vi "_LC Send Command.vi"(4 "VialNumber":i16=1, 5 "SparkParameters":T1={"PlatePosition"=1, "SampleColumn"=97, "TrayType"=3}, 6 "RackType":i32(ring) items=["RackSVial"=0, "RackLVial"=1, "RackSPeltier"=2, "RackLPeltier"=3, "RackSingleMTP"=4, "RackDualMTP"=5, "RackLL"=6, "Rack2"=17, "Rack1"=18, "Rack3"=19, "Rack4"=20, "Rack5"=21, "Rack6"=22, "Rack7"=23, "Rack12"=33, "Rack11"=34, "Rack13"=35, "Rack14"=36, "Rack15"=37, "Rack16"=38, "Rack17"=39, "Rack_2010A_15Standard"=49, "Rack_2010A_1Standard"=50, "Rack_2010A_4Standard"=51, "Rack_2010A_MTP96Standard"=52, "Rack_2010A_MTP384Standard"=53, "Rack_2010A_DW96Standard"=54, "Rack_2010A_DW384Standard"=55, "Rack_2010A_15Cooled"=65, "Rack_2010A_1Cooled"=66, "Rack_2010A_4Cooled"=67, "Rack_2010A_MTP96Cooled"=68, "Rack_2010A_MTP384Cooled"=69, "Rack_2010A_DW96Cooled"=70, "Rack_2010A_DW384Cooled"=71, "Rack_20A_RACKCHANGER"=72, "Rack12A"=80, "Rack14A"=81, "Rack8"=82, "Rack9"=83, "Rack10"=84, "Rack14DDW"=85, "Rack5U"=86, "Rack4U"=87, "ControlRack"=119, "RackNone"=136, "RackUnknown"=153], 7 "InjectionVolume":dbl=2.0, 8 "error in":errorcluster, 9 "Stream#":u8, 10 "Parameter":string, 11 "Command":T2) -> (0 "error out":errorcluster, 3 "Reply":string)   [LabVIEW 2015]
uses:
  Type/_LC Command.ctl
  Type/_Log Command.ctl
  _Global LC Driver.vi
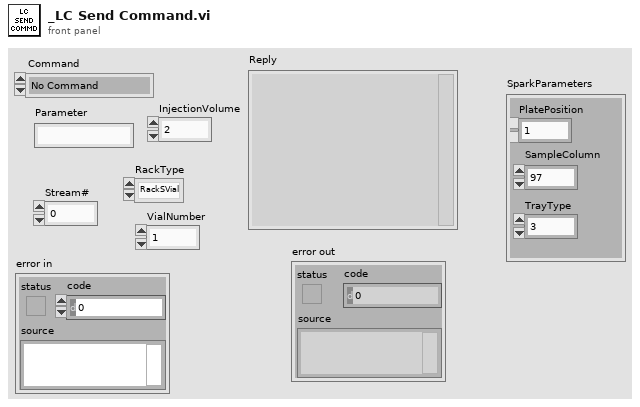
[diagram p1: front panel]
types:
  T1 = cluster{"PlatePosition":u8, "SampleColumn":u8, "TrayType":u8}
  T2 = typedef "_LC Command.ctl" = enum16{"No Command", "Initialize", "Get Configuration", "Get Status", "Get LC Method Contents", "Oven OnOff", "Pump OnOFF", "Rinse Autosampler", "Run Sample", "Set EnvParameters", "Set Method", "Start Equilibration", "Stop Run", "Get LastError", "Clear Error", "Close"}
  T3 = typedef "_Log Command.ctl" = enum16{"No Command", "Open", "Read", "Write", "Close", "Check Size"}
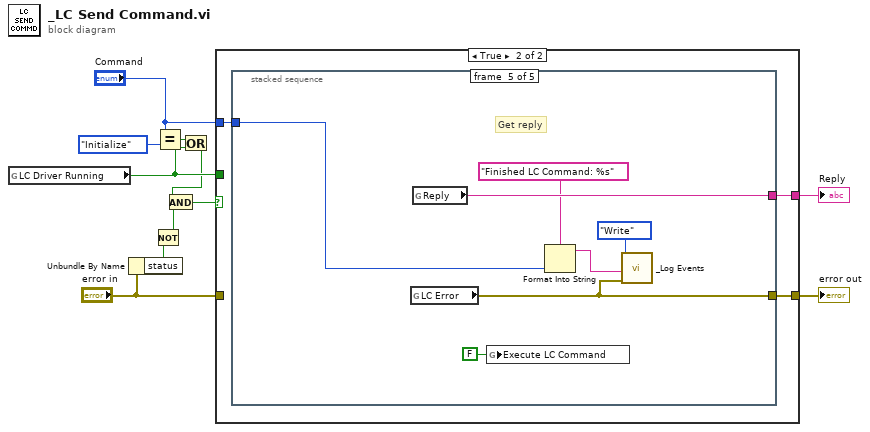
[diagram p0: block diagram]
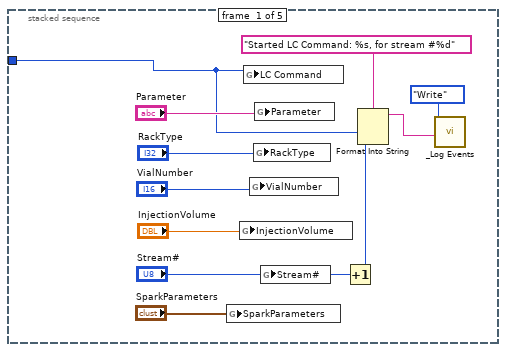
[diagram p3: hidden frame]
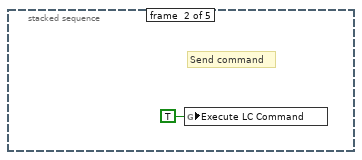
[diagram p4: hidden frame]
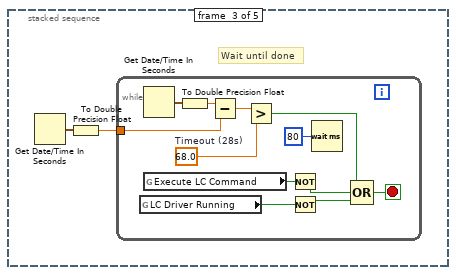
[diagram p5: hidden frame]
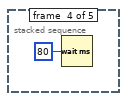
[diagram p6: hidden frame]
diagram:
  n1 = global read "_Global LC Driver.vi" "LC Driver Running"() -> (w2:bool)
  n2 = Unbundle By Name("error in") -> ("status"=w10:bool)
  n3 = Not(x=w10) -> (.not. x?=w9:bool)
  n4 = Equal?(x="Command", y=_LC_Command."Initialize") -> (x = y?=w3:bool)
  n5 = Or(x=w3, y=w2) -> (x .or. y?=w1:bool)
  n6 = And(x=w1, y=w9) -> (x .and. y?=w8:bool)
  n7 = case shown="True" w8 {
    tunnel: [w12 w15] -> w11
    tunnel: "error in" -> [w12 _]
    tunnel: "Command" -> [_ w14]
    tunnel: w2 -> [_ _]
    tunnel: [_ w13] -> w6
    frame False {
    }
    frame True {
      n8 = stacked-sequence {
        tunnel: [_ _ _ _ w44] -> w15
        tunnel: w14 -> [w22 _ _ _ w43]
        tunnel: [_ _ _ _ w48] -> w13
        frame #0 {
          n9 = global write "_Global LC Driver.vi" "SparkParameters"("SparkParameters") -> ()
          n10 = global write "_Global LC Driver.vi" "InjectionVolume"("InjectionVolume") -> ()
          n11 = global write "_Global LC Driver.vi" "LC Command"(w22) -> ()
          n12 = global write "_Global LC Driver.vi" "VialNumber"("VialNumber") -> ()
          n13 = global write "_Global LC Driver.vi" "RackType"("RackType") -> ()
          n14 = global write "_Global LC Driver.vi" "Parameter"("Parameter") -> ()
          n15 = global write "_Global LC Driver.vi" "Stream#"("Stream#") -> ()
          n16 = Increment(x="Stream#") -> (x+1=w16:u8)
          n17 = Format Into String(format string="Started LC Command: %s, for stream #%d", w22, w16) -> (resulting string=w20:string)  [unwired: 2 in, 1 out]
          n18 = call "_Log Events.vi"("Event"=w20, "Log Command"=_Log_Command."Write") -> ()  [unwired: 6 in, 2 out]
        }
        frame #1 {
          # "Send command"
          n19 = global write "_Global LC Driver.vi" "Execute LC Command"(TRUE ("Execute LC Command")) -> ()
        }
        frame #2 {
          # "Wait until done"
          n20 = Get Date/Time In Seconds() -> (seconds since 1Jan1904=w29:timestamp)
          n21 = To Double Precision Float(number=w29) -> (double precision float=w28:dbl)
          n22 = while {
            tunnel: w28 -> [w39]
            stop <- w37 stop-if-true
            w34 = 68.0  # Timeout (28s)
            n23 = global read "_Global LC Driver.vi" "LC Driver Running"() -> (w31:bool)
            n24 = Get Date/Time In Seconds() -> (seconds since 1Jan1904=w41:timestamp)
            n25 = global read "_Global LC Driver.vi" "Execute LC Command"() -> (w33:bool)
            n26 = To Double Precision Float(number=w41) -> (double precision float=w40:dbl)
            n27 = Subtract(x=w40, y=w39) -> (x-y=w38:dbl)
            n28 = Greater?(x=w38, y=w34) -> (0:w36:bool)
            n29 = Not(x=w33) -> (.not. x?=w32:bool)
            n30 = Not(x=w31) -> (.not. x?=w30:bool)
            n31 = Wait (ms)(milliseconds to wait=u32 80) -> ()  [unwired: 1 out]
            n32 = Compound Arithmetic op=OR(w36, w32, w30) -> (w37:bool)
          }
        }
        frame #3 {
          n33 = Wait (ms)(milliseconds to wait=u32 80) -> ()  [unwired: 1 out]
        }
        frame #4 {
          # "Get reply"
          n34 = global read "_Global LC Driver.vi" "LC Error"() -> (w44:errorcluster)
          n35 = global read "_Global LC Driver.vi" "Reply"() -> (w48:string)
          n36 = global write "_Global LC Driver.vi" "Execute LC Command"(FALSE ("Execute LC Command")) -> ()
          n37 = Format Into String(format string="Finished LC Command: %s", w43) -> (resulting string=w46:string)  [unwired: 2 in, 1 out]
          n38 = call "_Log Events.vi"("error in (no error)"=w44, "Event"=w46, "Log Command"=_Log_Command."Write") -> ()  [unwired: 5 in, 2 out]
        }
      }
    }
  }
  "error out" <- w11
  "Reply" <- w6
